vi "HXG2_LOAD Config File Values.vi"(8 "error in":errorcluster, 9 "All Ctrls Refs":refnum<vi>[](array[refnum]), 10 "All Bool Refs":refnum<vi>[](array[refnum])) -> (0 "error out":errorcluster, 3 "PID Gains Out":T1)   [LabVIEW 2012]
uses:
  Controls/HXG2_AirGly-Cluster.ctl
  Controls/UI/HXG2_UI_ControlSetAir.ctl
  Controls/UI/HXG2_UI_ControlSetGly.ctl
  PID/HXG2_Horizontal PID Control.ctl
  Modules/PID/HXG2pid.ctl
  Controls/HXG2_LiqHeat-Cascade.ctl
  Controls/HXG2_Aircool-Cascade.ctl
  <vilib>/Utility/file.llb/Read From Spreadsheet File (DBL).vi
panel:
  out "size(s) 2":i32
  out "size(s)":i32[](array[numeric])
  out "subarray":dbl[](array[numeric])
  out "Array":T2(array[cluster])
  out "Array Out":dbl[][](array[numeric])
  out "all rows":dbl[][](array[numeric]) format="%0.3f"
  out "PIDgains path":path
  out "appended path":path
  in  "AIR-GLY Cluster":T3 {"Liq Cluster"."Liq TEMP %" min=0.0 max=100.0 step=1.0 format="%#.1f"; "Liq Cluster"."Liq FLOW %" min=0.0 max=100.0 step=1.0 format="%#.1f"; "Liq Cluster"."TLiq °F" min=40.0 max=180.0 step=1.0 format="%#.1f"; "Liq Cluster"."Mdot lbm/hr" min=0.0 max=1000.0 step=1.0 format="%#.1f"; "Air Cluster"."Air TEMP %" min=0.0 max=100.0 step=1.0 format="%#.1f"; "Air Cluster"."Air FLOW %" min=0.0 max=100.0 step=1.0 format="%#.1f"; "Air Cluster"."Tair  °F" min=-5.0 max=100.0 step=1.0 format="%#.1f"; "Air Cluster"."CFMs" min=0.0 max=200.0 step=1.0 format="%#.1f"}
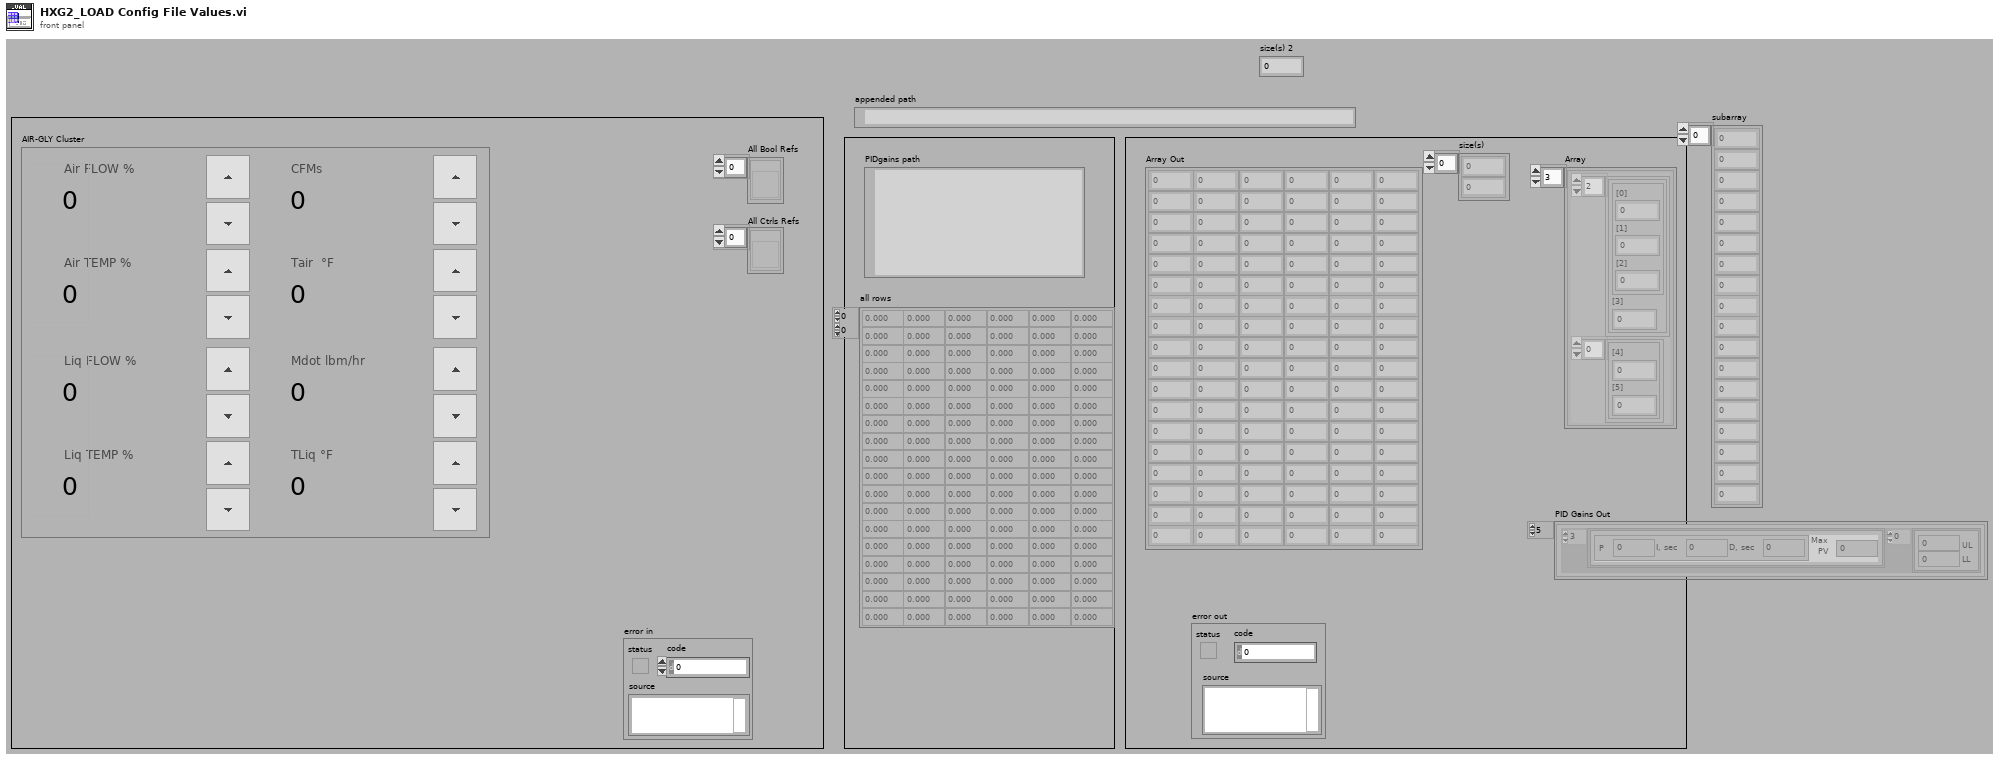
[diagram p1: front panel]
types:
  T1 = typedef "HXG2_Horizontal PID Control.ctl" = cluster{"GainsArray":cluster{"Gains 2":cluster{"P":dbl, "I, sec":dbl, "D, sec":dbl}, "Max\nPV":dbl}[], "UL-LL Array":cluster{"UL":dbl, "LL  ":dbl}[]}[]
  T2 = cluster{cluster{cluster{"[0]":dbl, "[1]":dbl, "[2]":dbl}, "[3]":dbl}[], cluster{"[4]":dbl, "[5]":dbl}[]}[]
  T3 = typedef "HXG2_AirGly-Cluster.ctl" = cluster{"Air Cluster":T4, "Liq Cluster":T5}
  T4 = typedef "HXG2_UI_ControlSetAir.ctl" = cluster{"Air FLOW %":dbl, "Air TEMP % ":dbl, "CFMs":dbl, "Tair  °F":dbl}
  T5 = typedef "HXG2_UI_ControlSetGly.ctl" = cluster{"Liq FLOW %":dbl, "Liq TEMP % ":dbl, "Mdot lbm/hr":dbl, "TLiq °F":dbl}
  T6 = cluster{cluster{"[0]":dbl, "[1]":dbl, "[2]":dbl}, "[3]":dbl}[]
  T7 = typedef "HXG2pid.ctl" = enum16{"Write PID Efforts", "Write PID On-Off", "Pass", "Write PID Refs", "Write PID Gains", "Wrt PID Resets"}
  T8 = typedef "HXG2_Aircool-Cascade.ctl" = cluster{"PID gains":cluster{"proportional gain (Kc)":dbl, "integral time (Ti, min)":dbl, "derivative time (Td, min)":dbl}, "output range":cluster{"output high":dbl, "output low":dbl}}
  T9 = typedef "HXG2_LiqHeat-Cascade.ctl" = cluster{"PID gains":cluster{"proportional gain (Kc)":dbl, "integral time (Ti, min)":dbl, "derivative time (Td, min)":dbl}, "output range":cluster{"output high":dbl, "output low":dbl}}
  T10 = cluster{"first row[0]":dbl, "first row[1]":dbl, "first row[2]":dbl, "first row[3]":dbl, "first row[4]":dbl, "first row[5]":dbl, "first row[6]":dbl, "first row[7]":dbl, "first row[8]":dbl, "first row[9]":dbl}
  T11 = cluster{"[0]":dbl, "[1]":dbl, "[2]":dbl, "[3]":dbl}
  T12 = cluster{"Boolean array[0]":bool, "Boolean array[1]":bool, "Boolean array[2]":bool, "Boolean array[3]":bool, "Boolean array[4]":bool, "Boolean array[5]":bool, "Boolean array[6]":bool, "Boolean array[7]":bool, "Boolean array[8]":bool, "Boolean array[9]":bool, "Boolean array[10]":bool, "Boolean array[11]":bool, "Boolean array[12]":bool, "Boolean array[13]":bool, "Boolean array[14]":bool, "Boolean array[15]":bool, "Boolean array[16]":bool, "Boolean array[17]":bool, "Boolean array[18]":bool, "Boolean array[19]":bool}
  T13 = cluster{cluster{cluster{"[0]":dbl, "[1]":dbl, "[2]":dbl}, "[3]":dbl}[], cluster{"[4]":dbl, "[5]":dbl}[]}
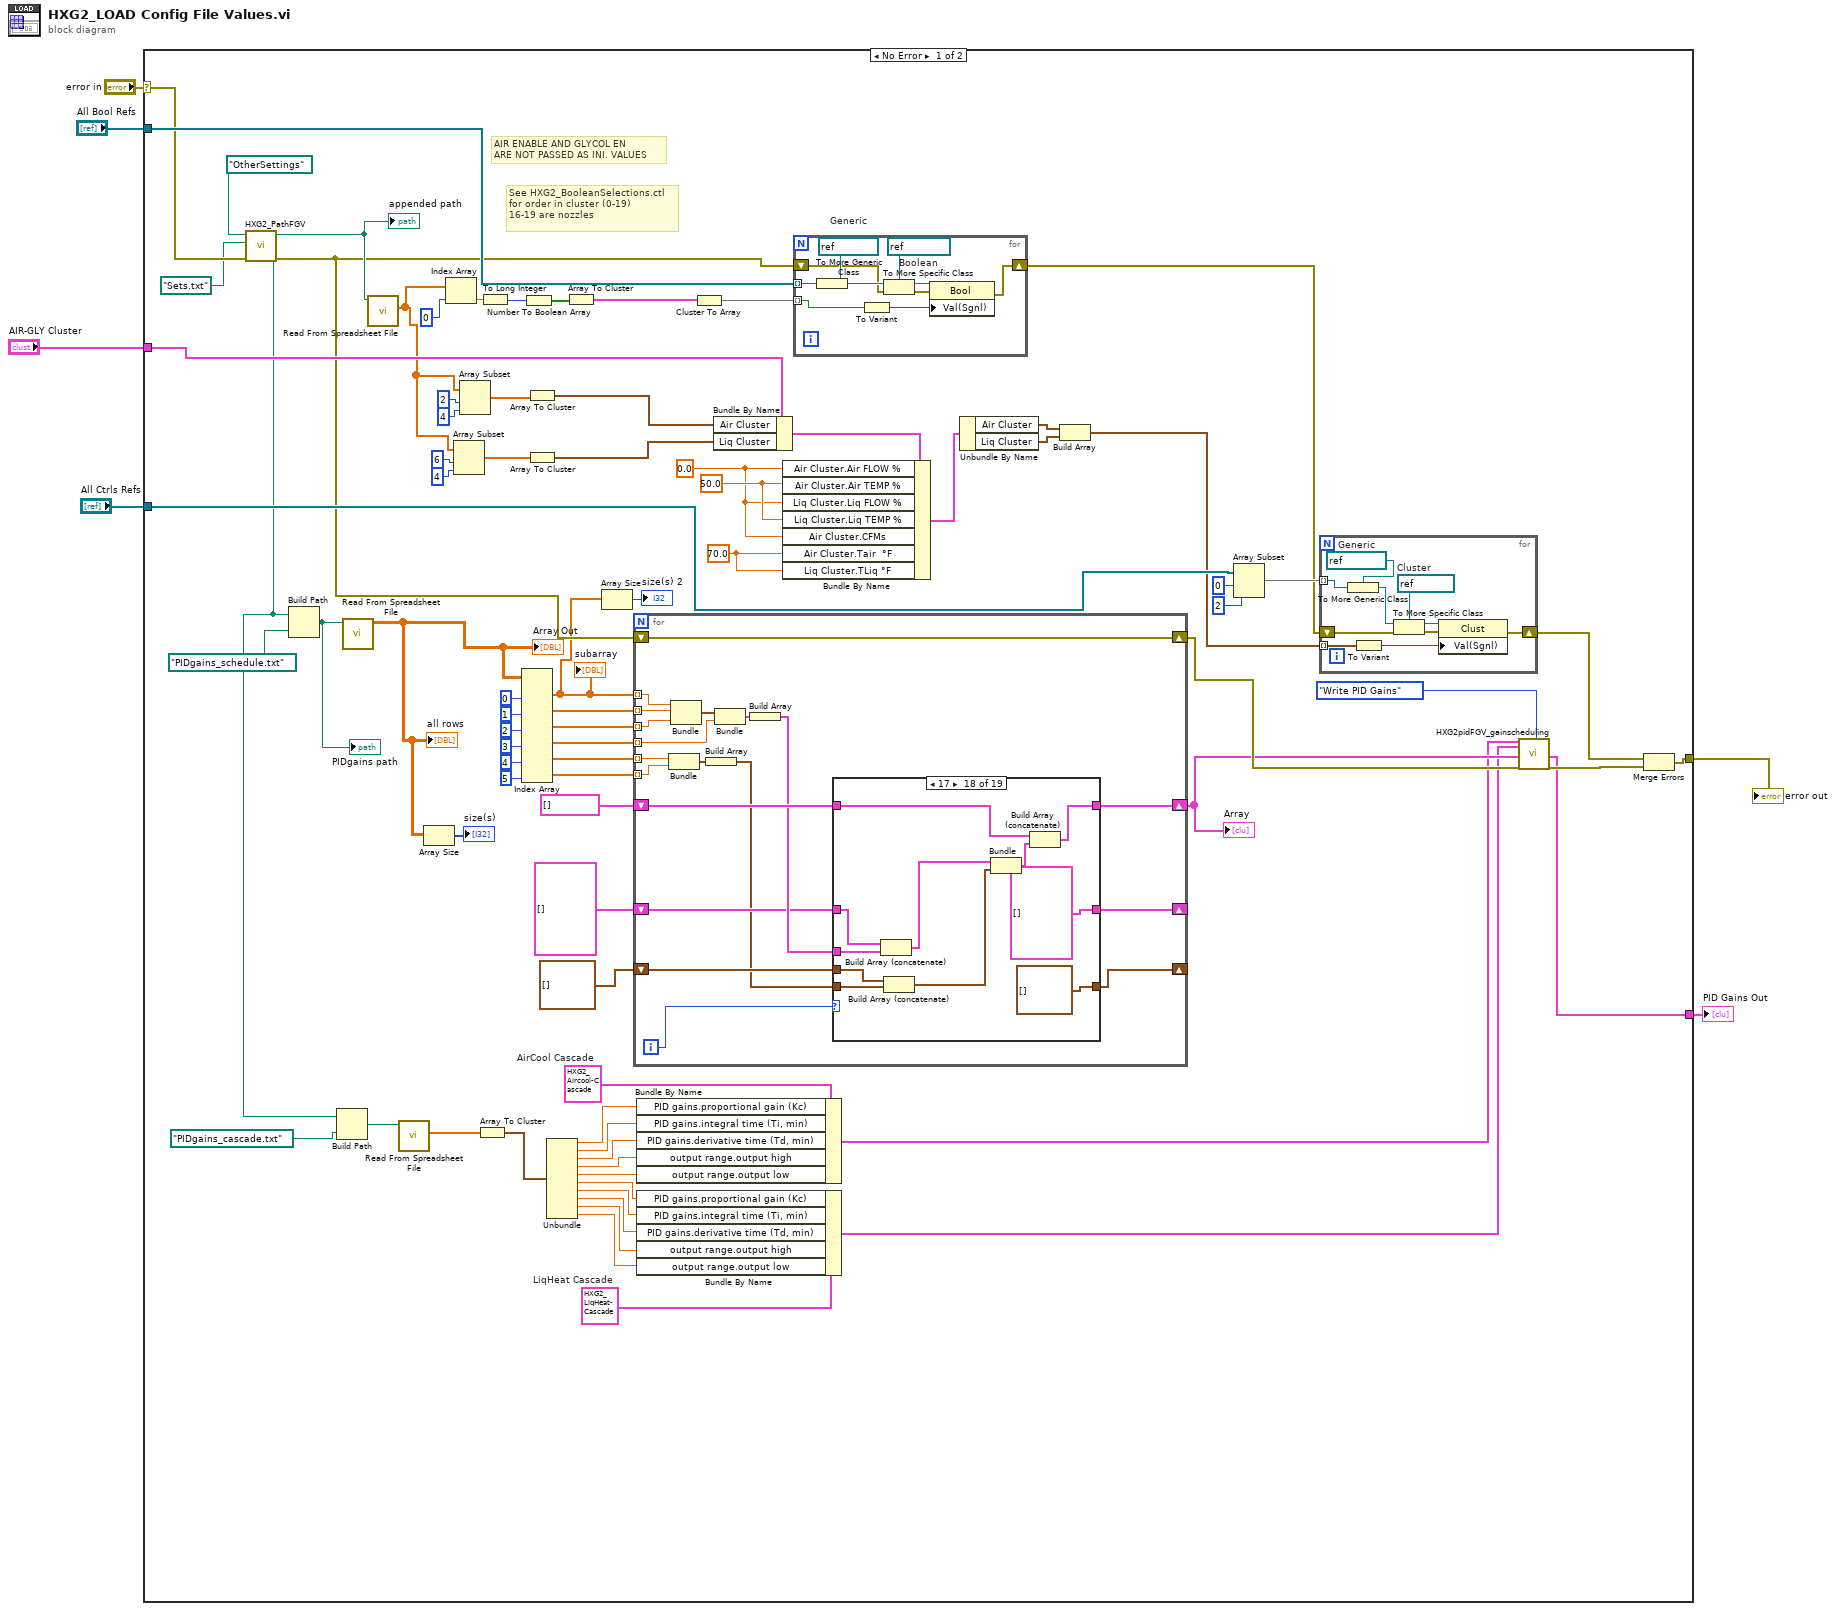
[diagram p0: block diagram]
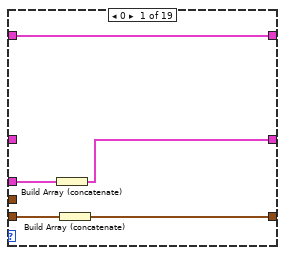
[diagram p2: hidden frame]
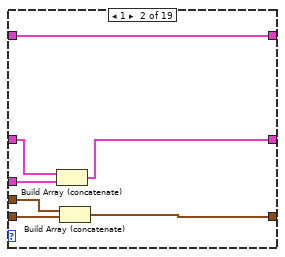
[diagram p3: hidden frame]
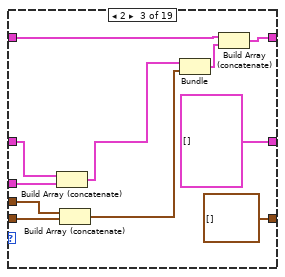
[diagram p4: hidden frame]
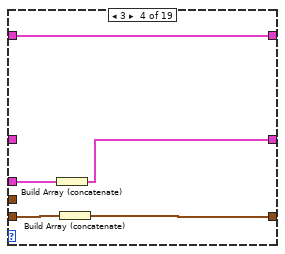
[diagram p5: hidden frame]
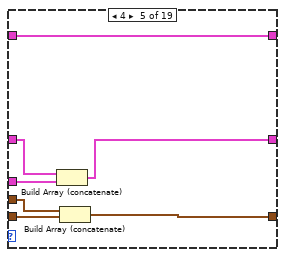
[diagram p6: hidden frame]
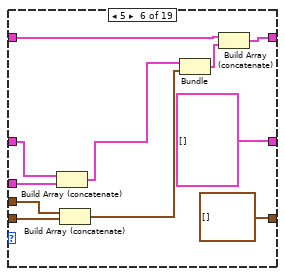
[diagram p7: hidden frame]
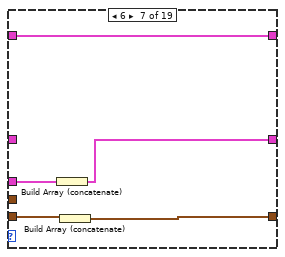
[diagram p8: hidden frame]
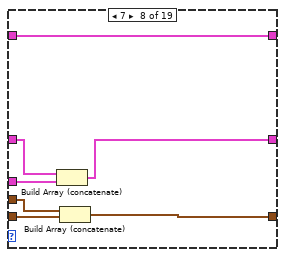
[diagram p9: hidden frame]
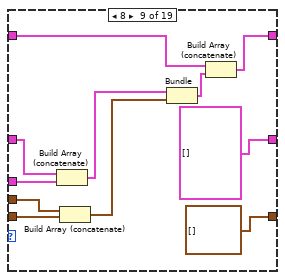
[diagram p10: hidden frame]
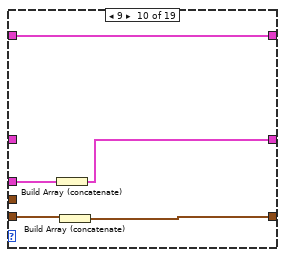
[diagram p11: hidden frame]
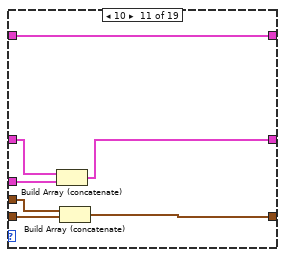
[diagram p12: hidden frame]
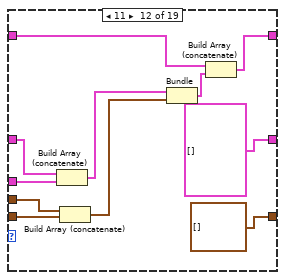
[diagram p13: hidden frame]
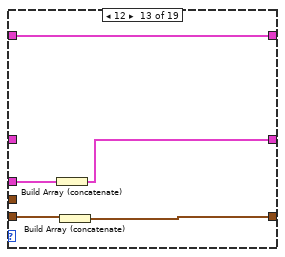
[diagram p14: hidden frame]
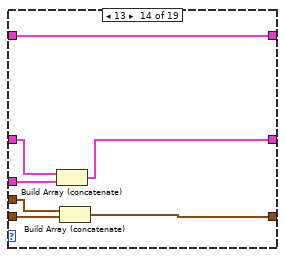
[diagram p15: hidden frame]
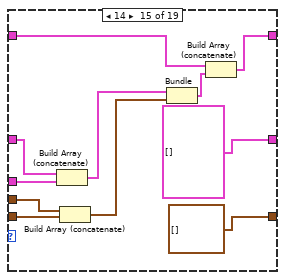
[diagram p16: hidden frame]
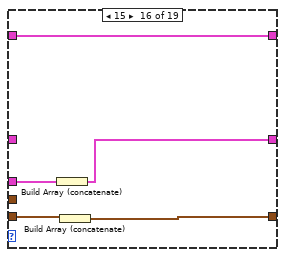
[diagram p17: hidden frame]
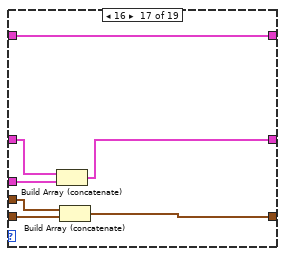
[diagram p18: hidden frame]
diagram:
  n1 = case shown="No Error" "error in" {
    selector: "error in" -> [w60 w268]
    tunnel: "All Ctrls Refs" -> [w78 _]
    tunnel: [w47 w268] -> w6
    tunnel: "All Bool Refs" -> [w64 _]
    tunnel: "AIR-GLY Cluster" -> [w77 _]
    tunnel: [w31 _] -> w1
    frame No Error {
      w21 = T8 {"PID gains"={"proportional gain (Kc)"=-1.15, "integral time (Ti, min)"=2.44, "derivative time (Td, min)"=0.0}, "output range"={"output high"=100.0, "output low"=10.0}}  # AirCool Cascade
      w14 = T9 {"PID gains"={"proportional gain (Kc)"=3.54, "integral time (Ti, min)"=46.25, "derivative time (Td, min)"=0.0}, "output range"={"output high"=100.0, "output low"=0.0}}  # LiqHeat Cascade
      w26 = 70.0 ("Air Cluster.Air FLOW %")
      w28 = 50.0 ("Air Cluster.Air FLOW %")
      w27 = 0.0 ("Air Cluster.Air FLOW %")
      # "See HXG2_BooleanSelections.ctl\nfor order in cluster (0-19)\n16-19 are nozzles"
      # "AIR ENABLE AND GLYCOL EN\nARE NOT PASSED AS INI. VALUES"
      n2 = call "HXG2_PathFGV.vi"("error in (no error)"=w60, "File Name"=path "Sets.txt", "Folder Name"=path "OtherSettings") -> ("error out"=w50:errorcluster, "Folder Path"=w25:path, "File path"=w57:path)  [unwired: 5 in, 1 out]
      "appended path" <- w57
      n3 = Build Path(base path=w25, name or relative path=path "PIDgains_schedule.txt") -> (appended path=w62:path)
      "PIDgains path" <- w62
      n4 = Build Path(base path=w25, name or relative path=path "PIDgains_cascade.txt") -> (appended path=w23:path)
      n5 = call-poly <vilib>:"Read From Spreadsheet File.vi"("file path (dialog if empty)"=w62) -> ("all rows"=w35:dbl[][])  [unwired: 6 in, 4 out]
      "all rows" <- w35
      "Array Out" <- w35
      n6 = call-poly <vilib>:"Read From Spreadsheet File.vi"("file path (dialog if empty)"=w57) -> ("first row"=w63:dbl[])  [unwired: 6 in, 4 out]
      n7 = call-poly <vilib>:"Read From Spreadsheet File.vi"("file path (dialog if empty)"=w23) -> ("first row"=w22:dbl[])  [unwired: 6 in, 4 out]
      n8 = Array Size(array=w35) -> (size(s)=→"size(s)":i32[])
      n9 = Index Array(array=w63, index=0) -> (element=w86:dbl)
      n10 = Array Subset(array=w63, index=6, length=4 ("index")) -> (w68:dbl[])
      n11 = Array Subset(array=w63, index=2, length=4 ("index")) -> (w69:dbl[])
      n12 = Array To Cluster(array=w22) -> (cluster=w20:T10)
      n13 = To Long Integer(number=w86) -> (32bit integer=w85:i32)
      n14 = Index Array(array=w35, index (col) #1=0 ("index (row)"), index (col) #2=1 ("index (row)"), index (col) #3=2 ("index (row)"), index (col) #4=3 ("index (row)"), index (col) #5=4 ("index (row)"), index (col) #6=5 ("index (row)")) -> (element #1=w33:dbl[], element #2=w55:dbl[], element #3=w54:dbl[], element #4=w53:dbl[], element #5=w52:dbl[], element #6=w51:dbl[])  [unwired: 6 in]
      "subarray" <- w33
      n15 = Number To Boolean Array(number=w85) -> (Boolean array=w84:bool[])
      n16 = Array To Cluster(array=w69) -> (cluster=w67:T11)
      n17 = Array To Cluster(array=w68) -> (cluster=w66:T11)
      n18 = Unbundle(w20) -> ("first row[0]"=w19:dbl, "first row[1]"=w18:dbl, "first row[2]"=w17:dbl, "first row[3]"=w16:dbl, "first row[4]"=w15:dbl, "first row[5]"=w13:dbl, "first row[6]"=w12:dbl, "first row[7]"=w11:dbl, "first row[8]"=w10:dbl, "first row[9]"=w9:dbl)
      n19 = Array To Cluster(array=w84) -> (cluster=w82:T12)
      n20 = Array Size(array=w33) -> (size(s)=→"size(s) 2":i32)
      n21 = for {
        tunnel: w33 -> [w105] mode=indexing
        tunnel: w55 -> [w106] mode=indexing
        tunnel: w54 -> [w104] mode=indexing
        tunnel: w53 -> [w100] mode=indexing
        tunnel: w52 -> [w103] mode=indexing
        tunnel: w51 -> [w102] mode=indexing
        shift-right: [w99] -> w37
        shift-left: w50 -> [w99]
        shift-right: [w88] -> w36
        shift-left: T2 [] -> [w98]
        shift-right: [w91] -> _
        shift-left: T6 [] ("appended array") -> [w92]
        shift-right: [w90] -> _
        shift-left: cluster{"[4]":dbl, "[5]":dbl}[] [] ("appended array") -> [w94]
        i -> [w93]
        n22 = Bundle(w103, w102) -> (w96:cluster{dbl, dbl})  [unwired: 1 in]
        n23 = Bundle(w105, w106, w104) -> (w101:cluster{dbl, dbl, dbl})  [unwired: 1 in]
        n24 = Build Array(w96) -> (w89:cluster{dbl, dbl}[])
        n25 = Bundle(w101, w100) -> (w97:cluster{cluster{dbl, dbl, dbl}, dbl})  [unwired: 1 in]
        n26 = Build Array(w97) -> (w95:cluster{cluster{dbl, dbl, dbl}, dbl}[])
        n27 = case shown="17" w93 {
          tunnel: w95 -> [w111 w118 w129 w134 w141 w152 w157 w164 w175 w180 w187 w198 w203 w210 w221 w226 w233 w244 _]
          tunnel: w89 -> [w110 w117 w128 w133 w140 w151 w156 w163 w174 w179 w186 w197 w202 w209 w220 w225 w232 w243 _]
          tunnel: w94 -> [_ w116 w127 _ w135 w150 _ w158 w173 _ w181 w196 _ w204 w219 _ w227 w242 w247]
          tunnel: [w109 w115 T6 [] ("appended array") w132 w139 T6 [] ("appended array") w155 w162 T6 [] ("appended array") w178 w185 T6 [] ("appended array") w201 w208 T6 [] ("appended array") w224 w231 T6 [] ("appended array") w245] -> w91
          tunnel: [w108 w114 cluster{"[4]":dbl, "[5]":dbl}[] [] ("appended array") w131 w138 cluster{"[4]":dbl, "[5]":dbl}[] [] ("appended array") w154 w161 cluster{"[4]":dbl, "[5]":dbl}[] [] ("appended array") w177 w184 cluster{"[4]":dbl, "[5]":dbl}[] [] ("appended array") w200 w207 cluster{"[4]":dbl, "[5]":dbl}[] [] ("appended array") w223 w230 cluster{"[4]":dbl, "[5]":dbl}[] [] ("appended array") w247] -> w90
          tunnel: w98 -> [w107 w113 w125 w130 w137 w147 w153 w160 w168 w176 w183 w191 w199 w206 w214 w222 w229 w237 w246]
          tunnel: [w107 w113 w123 w130 w137 w145 w153 w160 w167 w176 w183 w190 w199 w206 w213 w222 w229 w236 w246] -> w88
          tunnel: w92 -> [_ w112 w122 _ w136 w144 _ w159 w172 _ w182 w195 _ w205 w218 _ w228 w241 w245]
          frame 0 {
            n28 = Build Array (concatenate)(w111) -> (w109:cluster{cluster{dbl, dbl, dbl}, dbl}[])
            n29 = Build Array (concatenate)(w110) -> (w108:cluster{dbl, dbl}[])
          }
          frame 1 {
            n30 = Build Array (concatenate)(w112, w118) -> (w115:T6)
            n31 = Build Array (concatenate)(w116, w117) -> (w114:cluster{"[4]":dbl, "[5]":dbl}[])
          }
          frame 2 {
            n32 = Build Array (concatenate)(w122, w129) -> (w126:T6)
            n33 = Build Array (concatenate)(w127, w128) -> (w120:cluster{"[4]":dbl, "[5]":dbl}[])
            n34 = Bundle(w126, w120) -> (w124:T13)  [unwired: 1 in]
            n35 = Build Array (concatenate)(w125, w124) -> (w123:T2)
          }
          frame 3 {
            n36 = Build Array (concatenate)(w134) -> (w132:cluster{cluster{dbl, dbl, dbl}, dbl}[])
            n37 = Build Array (concatenate)(w133) -> (w131:cluster{dbl, dbl}[])
          }
          frame 4 {
            n38 = Build Array (concatenate)(w136, w141) -> (w139:T6)
            n39 = Build Array (concatenate)(w135, w140) -> (w138:cluster{"[4]":dbl, "[5]":dbl}[])
          }
          frame 5 {
            n40 = Build Array (concatenate)(w144, w152) -> (w149:T6)
            n41 = Build Array (concatenate)(w150, w151) -> (w148:cluster{"[4]":dbl, "[5]":dbl}[])
            n42 = Bundle(w149, w148) -> (w146:T13)  [unwired: 1 in]
            n43 = Build Array (concatenate)(w147, w146) -> (w145:T2)
          }
          frame 6 {
            n44 = Build Array (concatenate)(w157) -> (w155:cluster{cluster{dbl, dbl, dbl}, dbl}[])
            n45 = Build Array (concatenate)(w156) -> (w154:cluster{dbl, dbl}[])
          }
          frame 7 {
            n46 = Build Array (concatenate)(w159, w164) -> (w162:T6)
            n47 = Build Array (concatenate)(w158, w163) -> (w161:cluster{"[4]":dbl, "[5]":dbl}[])
          }
          frame 8 {
            n48 = Build Array (concatenate)(w172, w175) -> (w170:T6)
            n49 = Build Array (concatenate)(w173, w174) -> (w169:cluster{"[4]":dbl, "[5]":dbl}[])
            n50 = Bundle(w170, w169) -> (w171:T13)  [unwired: 1 in]
            n51 = Build Array (concatenate)(w168, w171) -> (w167:T2)
          }
          frame 9 {
            n52 = Build Array (concatenate)(w180) -> (w178:cluster{cluster{dbl, dbl, dbl}, dbl}[])
            n53 = Build Array (concatenate)(w179) -> (w177:cluster{dbl, dbl}[])
          }
          frame 10 {
            n54 = Build Array (concatenate)(w182, w187) -> (w185:T6)
            n55 = Build Array (concatenate)(w181, w186) -> (w184:cluster{"[4]":dbl, "[5]":dbl}[])
          }
          frame 11 {
            n56 = Build Array (concatenate)(w195, w198) -> (w193:T6)
            n57 = Build Array (concatenate)(w196, w197) -> (w192:cluster{"[4]":dbl, "[5]":dbl}[])
            n58 = Bundle(w193, w192) -> (w194:T13)  [unwired: 1 in]
            n59 = Build Array (concatenate)(w191, w194) -> (w190:T2)
          }
          frame 12 {
            n60 = Build Array (concatenate)(w203) -> (w201:cluster{cluster{dbl, dbl, dbl}, dbl}[])
            n61 = Build Array (concatenate)(w202) -> (w200:cluster{dbl, dbl}[])
          }
          frame 13 {
            n62 = Build Array (concatenate)(w205, w210) -> (w208:T6)
            n63 = Build Array (concatenate)(w204, w209) -> (w207:cluster{"[4]":dbl, "[5]":dbl}[])
          }
          frame 14 {
            n64 = Build Array (concatenate)(w218, w221) -> (w216:T6)
            n65 = Build Array (concatenate)(w219, w220) -> (w215:cluster{"[4]":dbl, "[5]":dbl}[])
            n66 = Bundle(w216, w215) -> (w217:T13)  [unwired: 1 in]
            n67 = Build Array (concatenate)(w214, w217) -> (w213:T2)
          }
          frame 15 {
            n68 = Build Array (concatenate)(w226) -> (w224:cluster{cluster{dbl, dbl, dbl}, dbl}[])
            n69 = Build Array (concatenate)(w225) -> (w223:cluster{dbl, dbl}[])
          }
          frame 16 {
            n70 = Build Array (concatenate)(w228, w233) -> (w231:T6)
            n71 = Build Array (concatenate)(w227, w232) -> (w230:cluster{"[4]":dbl, "[5]":dbl}[])
          }
          frame 17 {
            n72 = Build Array (concatenate)(w241, w244) -> (w239:T6)
            n73 = Build Array (concatenate)(w242, w243) -> (w238:cluster{"[4]":dbl, "[5]":dbl}[])
            n74 = Bundle(w239, w238) -> (w240:T13)  [unwired: 1 in]
            n75 = Build Array (concatenate)(w237, w240) -> (w236:T2)
          }
          frame Default {
          }
        }
      }
      "Array" <- w36
      n76 = Bundle By Name(cluster=w21, "PID gains.proportional gain (Kc)"=w19, "PID gains.integral time (Ti, min)"=w18, "PID gains.derivative time (Td, min)"=w17, "output range.output high"=w16, "output range.output low"=w15) -> (w8:T8)
      n77 = Bundle By Name(cluster=w14, "PID gains.proportional gain (Kc)"=w13, "PID gains.integral time (Ti, min)"=w12, "PID gains.derivative time (Td, min)"=w11, "output range.output high"=w10, "output range.output low"=w9) -> (w7:T9)
      n78 = Cluster To Array(cluster=w82) -> (array=w83:bool[])
      n79 = Bundle By Name(cluster=w77, "Air Cluster"=w67, "Liq Cluster"=w66) -> (w30:T3)
      n80 = Bundle By Name(cluster=w30, "Air Cluster.Air FLOW %"=w27, "Air Cluster.Air TEMP %"=w28, "Liq Cluster.Liq FLOW %"=w27, "Liq Cluster.Liq TEMP %"=w28, "Air Cluster.CFMs"=w27, "Air Cluster.Tair  °F"=w26, "Liq Cluster.TLiq °F"=w26) -> (w29:T3)
      n81 = for {
        shift-right: [w256] -> w65
        shift-left: w50 -> [w252]
        tunnel: w83 -> [w249] mode=indexing
        tunnel: w64 -> [w257] mode=indexing
        w251 = refnum<vi> refnum  # Boolean
        w254 = refnum<vi> refnum  # Generic
        n82 = To More Generic Class(target class=w254, reference=w257) -> (generic class reference=w255:refnum<vi>)
        n83 = To Variant(anything=w249) -> (Variant=w248:variant)
        n84 = To More Specific Class(target class=w251, reference=w255, error in=w252) -> (specific class reference=w253:refnum<vi>, error out=w250:errorcluster)
        n85 = property class="Bool"(reference=w253, error in=w250, "Val(Sgnl)"=w248) -> (error out=w256:errorcluster)  [unwired: 1 out]
      }
      n86 = Unbundle By Name(w29) -> ("Air Cluster"=w75:T4, "Liq Cluster"=w76:T5)
      n87 = Build Array(w75, w76) -> (w74:T5[])
      n88 = Array Subset(array=w78, index=0, length=2) -> (w79:refnum<vi>[])
      n89 = for {
        shift-right: [w267] -> w49
        shift-left: w65 -> [w260]
        tunnel: w79 -> [w265] mode=indexing
        tunnel: w74 -> [w258] mode=indexing
        w261 = refnum<vi> refnum  # Cluster
        w263 = refnum<vi> refnum  # Generic
        n90 = To More Generic Class(target class=w263, reference=w265) -> (generic class reference=w264:refnum<vi>)
        n91 = To Variant(anything=w258) -> (Variant=w266:variant)
        n92 = To More Specific Class(target class=w261, reference=w264, error in=w260) -> (specific class reference=w262:refnum<vi>, error out=w259:errorcluster)
        n93 = property class="Clust"(reference=w262, error in=w259, "Val(Sgnl)"=w266) -> (error out=w267:errorcluster)  [unwired: 1 out]
      }
      n94 = call "HXG2pidFGV_gainscheduling.vi"("AirCool Cascade"=w8, "LiqHeat Cascade"=w7, "PID gains in"=w36, "error in (no error)"=w37, "PIDfgvCtrl"=HXG2pid."Write PID Gains") -> ("PID Gains Out"=w31:T1, "error out"=w48:errorcluster)  [unwired: 6 in, 7 out]
      n95 = Merge Errors(w49, w48) -> (w47:errorcluster)
    }
    frame Error {
    }
  }
  "error out" <- w6
  "PID Gains Out" <- w1
